vi "PracticaTemperatura.vi"() -> ()   [LabVIEW 2014]
uses:
  <vilib>/Instr/_visa.llb/VISA Configure Serial Port (Instr).vi
panel:
  in  "Tab Control":enum32{"Temperatura", "Graficas"}(tab)
  in  "VISA resource name":refnum<visa-resource-name>
  in  "baud rate (9600)":u32=9600
  in  "Detener Todo":bool
  out "ADC NTC":i32
  out "ADC LM35 R":i32
  out "ADC LM35 L":i32
  out "LM35 R":dbl(slide) scale=0.0..100.0
  out "LM35 L":dbl(slide) scale=0.0..100.0
  out "NTC":dbl(slide) scale=0.0..100.0
  in  "Detenar Grafica":bool
  in  "Inicio":bool
  out "Waveform Chart":dbl[][](graph)
  out "R":dbl
  out "L":dbl
  out "V":dbl
  out "ln(x)":dbl
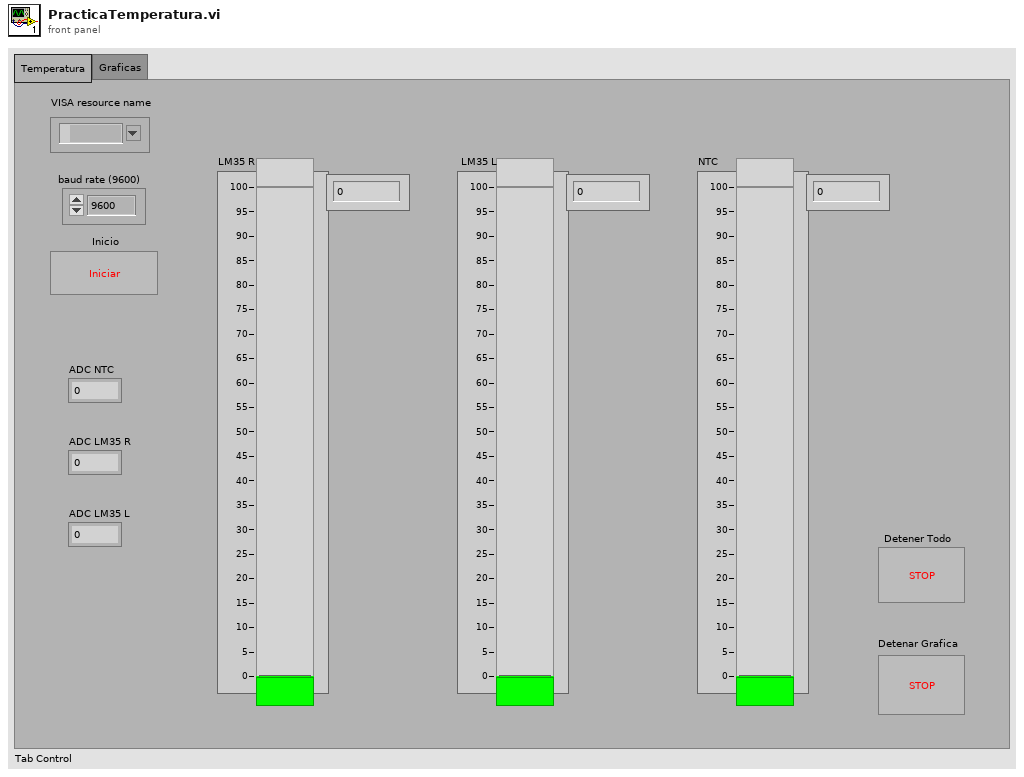
[diagram p1: front panel]
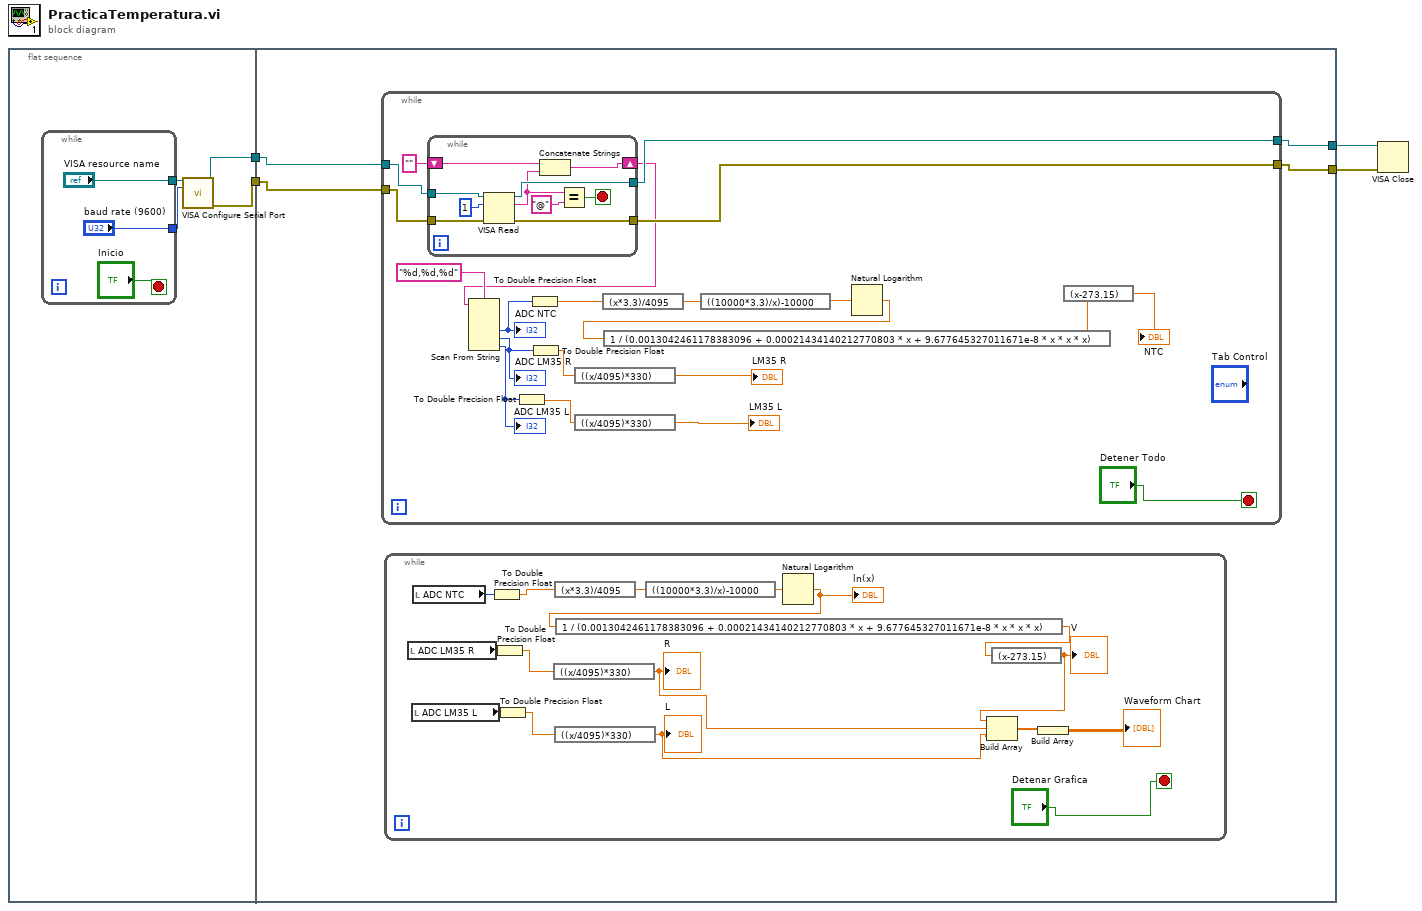
[diagram p0: block diagram]
diagram:
  n1 = flat-sequence {
    tunnel: [w8] -> w4
    tunnel: [w7] -> w3
    tunnel: w4 -> [w14]
    tunnel: w3 -> [w15]
    tunnel: [w13] -> w2
    tunnel: [w12] -> w1
    frame #0 {
      n2 = while {
        tunnel: ["baud rate (9600)"] -> w6
        tunnel: ["VISA resource name"] -> w5
        stop <- "Inicio" stop-if-true
      }
      n3 = call-poly "VISA Configure Serial Port"("VISA resource name"=w5, "baud rate (9600)"=w6) -> ("VISA resource name out"=w7:refnum<visa-resource-name>, "error out"=w8:errorcluster)  [unwired: 12 in]
    }
    frame #1 {
      n4 = while {
        tunnel: w15 -> [w52]
        tunnel: w14 -> [w51]
        tunnel: [w49] -> w13
        tunnel: [w48] -> w12
        stop <- "Detener Todo" stop-if-true
        n5 = while {
          tunnel: w52 -> [w62]
          tunnel: w51 -> [w61]
          tunnel: [w59] -> w49
          tunnel: [w58] -> w48
          shift-right: [w55] -> w33
          shift-left: "" -> [w54]
          stop <- w56 stop-if-true
          n6 = VISA Read(VISA resource name=w62, byte count=u32 1, error in (no error)=w61) -> (VISA resource name out=w59:refnum<visa-resource-name>, read buffer=w53:string, error out=w58:errorcluster)  [unwired: 1 out]
          n7 = Concatenate Strings(w54, w53) -> (w55:string)
          n8 = Equal?(x=w53, y="@") -> (x = y?=w56:bool)
        }
        n9 = Scan From String(format string="%d,%d,%d", input string=w33) -> (output 1=w41:i32, output 2=w45:i32, output 3=w46:i32)  [unwired: 5 in, 3 out]
        "ADC NTC" <- w41
        "ADC LM35 R" <- w45
        "ADC LM35 L" <- w46
        n10 = To Double Precision Float(number=w46) -> (double precision float=w34:dbl)
        n11 = To Double Precision Float(number=w41) -> (double precision float=w40:dbl)
        n12 = To Double Precision Float(number=w45) -> (double precision float=w44:dbl)
        n13 = expression code="((x/4095)*330)"(w44) -> (→"LM35 R":dbl)
        n14 = expression code="((x/4095)*330)"(w34) -> (→"LM35 L":dbl)
        n15 = expression code="(x*3.3)/4095"(w40) -> (w39:dbl)
        n16 = expression code="((10000*3.3)/x)-10000"(w39) -> (w38:dbl)
        n17 = Natural Logarithm(1:w38) -> (0:w37:dbl)
        n18 = expression code="1 / (0.0013042461178383096 + 0.00021434140212770803 * x + 9.677645327011671e-8 * x * x * x)"(w37) -> (w36:dbl)
        n19 = expression code="(x-273.15)"(w36) -> (→"NTC":dbl)
      }
      n20 = while {
        stop <- "Detenar Grafica" stop-if-true
        n21 = local read "ADC LM35 R"() -> (w30:i32)
        n22 = local read "ADC LM35 L"() -> (w29:i32)
        n23 = local read "ADC NTC"() -> (w31:i32)
        n24 = To Double Precision Float(number=w31) -> (double precision float=w26:dbl)
        n25 = To Double Precision Float(number=w30) -> (double precision float=w28:dbl)
        n26 = To Double Precision Float(number=w29) -> (double precision float=w27:dbl)
        n27 = expression code="((x/4095)*330)"(w28) -> (w21:dbl)
        "R" <- w21
        n28 = expression code="(x*3.3)/4095"(w26) -> (w25:dbl)
        n29 = expression code="((x/4095)*330)"(w27) -> (w20:dbl)
        "L" <- w20
        n30 = expression code="((10000*3.3)/x)-10000"(w25) -> (w24:dbl)
        n31 = Natural Logarithm(1:w24) -> (0:w23:dbl)
        "ln(x)" <- w23
        n32 = expression code="1 / (0.0013042461178383096 + 0.00021434140212770803 * x + 9.677645327011671e-8 * x * x * x)"(w23) -> (w22:dbl)
        n33 = expression code="(x-273.15)"(w22) -> (w18:dbl)
        "V" <- w18
        n34 = Build Array(w18, w21, w20) -> (w19:dbl[])
        n35 = Build Array(w19) -> (→"Waveform Chart":dbl[][])
      }
    }
  }
  n36 = VISA Close(VISA resource name=w2, error in (no error)=w1) -> ()  [unwired: 1 out]
